vi "OnDataDrag.vi"(0 "XRef":T13, 1 "Point":T11, 2 "String":T5, 3 "Path":T10, 4 "ProjectItemRefs":T8, 5 "GObjRefs":T6, 6 "State In":T1) -> (14 "Reply":T4, 15 "Fatal Error Out":T3, 16 "State Out":T1)   [LabVIEW 2018, in "RetryNode.xnode"]
uses:
  RetryNode.xnode
  <vilib>/XNodeSupport/XNodeXNodeRef.ctl
  <vilib>/XNodeSupport/XNodePoint.ctl
  <vilib>/XNodeSupport/XNodeInt.ctl
  <vilib>/XNodeSupport/XNodeString.ctl
  <vilib>/XNodeSupport/XNodePath.ctl
  <vilib>/XNodeSupport/XNodeProjItemRefArray.ctl
  <vilib>/XNodeSupport/XNodeProjItemRef.ctl
  <vilib>/XNodeSupport/XNodeGObjRefArray.ctl
  <vilib>/XNodeSupport/XNodeGObjRef.ctl
  State.ctl
  <vilib>/Utility/miscctls.llb/LVRectTypeDef.ctl
  <vilib>/XNodeSupport/XNodeStringArray.ctl
  <vilib>/XNodeSupport/XNodeErrorCluster.ctl
  <vilib>/XNodeSupport/NI_XNodeSupport.lvlib
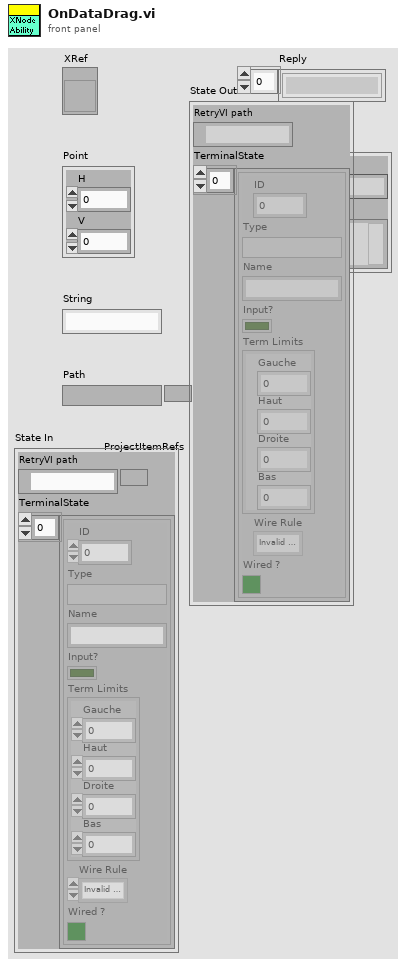
[diagram p1: front panel]
types:
  T1 = typedef "RetryNode.xnode/State.ctl" = cluster{"RetryVI path":path, "TerminalState":cluster{"ID":i32, "Type":variant, "Name":string, "Input?":bool, "Term Limits":T2, "Wire Rule":enum16{"Invalid Wire Rule", "Required", "Recommended", "Optional", "Dynamic Dispatch"}, "Wired ?":bool}[]}
  T2 = typedef "LVRectTypeDef.ctl" = cluster{"Left":i16, "Top":i16, "Right":i16, "Bottom":i16}
  T3 = typedef "NI_XNodeSupport.lvlib/XNodeErrorCluster.ctl" = errorcluster
  T4 = typedef "NI_XNodeSupport.lvlib/XNodeStringArray.ctl" = T5[]
  T5 = typedef "NI_XNodeSupport.lvlib/XNodeString.ctl" = string
  T6 = typedef "NI_XNodeSupport.lvlib/XNodeGObjRefArray.ctl" = T7[]
  T7 = typedef "NI_XNodeSupport.lvlib/XNodeGObjRef.ctl" = refnum<vi>
  T8 = typedef "NI_XNodeSupport.lvlib/XNodeProjItemRefArray.ctl" = T9[]
  T9 = typedef "NI_XNodeSupport.lvlib/XNodeProjItemRef.ctl" = refnum<vi>
  T10 = typedef "NI_XNodeSupport.lvlib/XNodePath.ctl" = path
  T11 = typedef "NI_XNodeSupport.lvlib/XNodePoint.ctl" = cluster{"H":T12, "V":T12}
  T12 = typedef "NI_XNodeSupport.lvlib/XNodeInt.ctl" = i32
  T13 = typedef "NI_XNodeSupport.lvlib/XNodeXNodeRef.ctl" = refnum<vi>
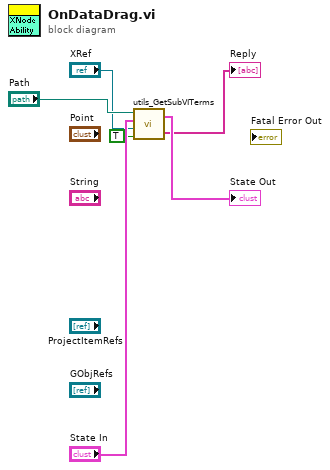
[diagram p0: block diagram]
diagram:
  n1 = call "utils_GetSubVITerms.vi"("Drop VI"=TRUE, "XRef"="XRef", "State In"="State In", "Path"="Path") -> ("Reply"=→"Reply":string[], "State Out"=→"State Out":T1)
